vi "fgv-GlobalCacher.vi"(6 "Boolean":bool, 8 "error in (no error)":errorcluster, 11 "Variant (in)":variant) -> (0 "error out":errorcluster, 3 "Variant":variant)   [LabVIEW 2017, in "ObjectCacherAPI.lvlib"]
uses:
  ObjectCacherAPI.lvlib
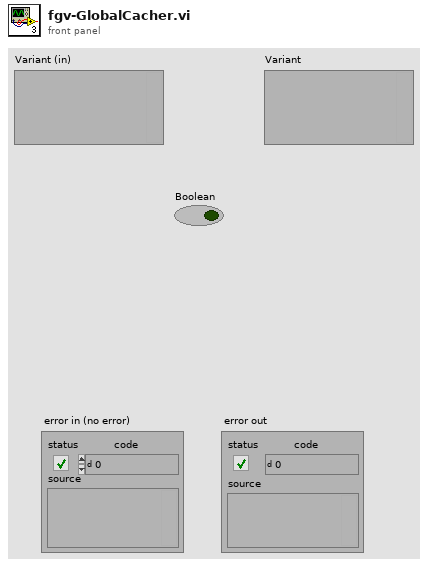
[diagram p1: front panel]
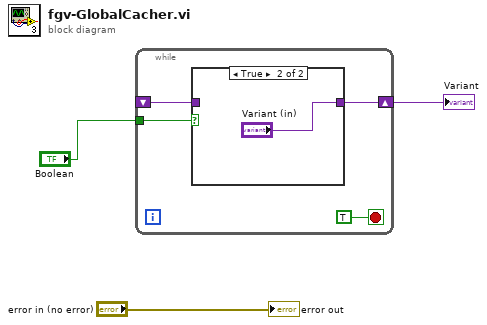
[diagram p0: block diagram]
diagram:
  n1 = while {
    shift-right: [w6] -> w3
    shift-left: _ -> [w5]
    tunnel: "Boolean" -> [w4]
    stop <- TRUE stop-if-true
    n2 = case shown="True" w4 {
      tunnel: [w8 "Variant (in)"] -> w6
      tunnel: w5 -> [w8 _]
      frame False {
      }
      frame True {
      }
    }
  }
  "Variant" <- w3
  "error out" <- "error in (no error)"
